vi "Do.vi"(8 "error in (no error)":errorcluster, 10 "Actor in":refnum<class "Actor.lvclass">, 11 "Launch Feature Test View Msg in":refnum<class "Launch Feature Test View Msg.lvclass">) -> (0 "error out":errorcluster, 2 "Actor out":refnum<class "Actor.lvclass">)   [LabVIEW 2023, in "Example Event Actors.lvlib" / "Example Controller Actor.lvlib" / "Launch Feature Test View Msg.lvclass"]
doc: "(<B>Filename</B>: Actor Framework.lvlib:Message.lvclass:Do.vi)\n\nDefines what a message does when it is received by an actor. Generally, a message instructs an actor to invoke one of its methods. By default, this method does nothing. A child class must override it to define behavior. Create a child class by using the Actor Framework Message Maker dialog box."
uses:
  Launch Feature Test View Msg.lvclass
  <vilib>/ActorFramework/Actor/Actor.lvclass
  Example Controller Actor/Example Controller Actor.lvclass
  Launch Feature Test View Msg.lvclass/Launch Feature Test View Msg.ctl
  C:/Projects/Shared Libraries/Event Actors/Examples/Timed Loop Controller/Timed Loop Controller/Timed Loop Controller.lvclass
  C:/Projects/Shared Libraries/Event Actors/Controller Actor/Controller Actor.lvclass
  C:/Program Files/National Instruments/LabVIEW 2023/vi.lib/ActorFramework/Actor/Actor.lvclass
  C:/Projects/Hardware Controller/Source/LSI Hardware Controller/View Interface/IView.lvclass
  C:/Projects/Shared Libraries/Event Actors/Examples/Example Controller Actor/Example Controller Actor/Example Controller Actor.lvclass
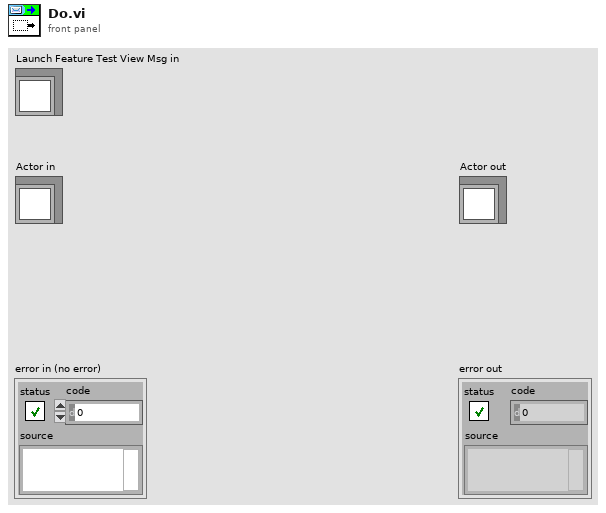
[diagram p1: front panel]
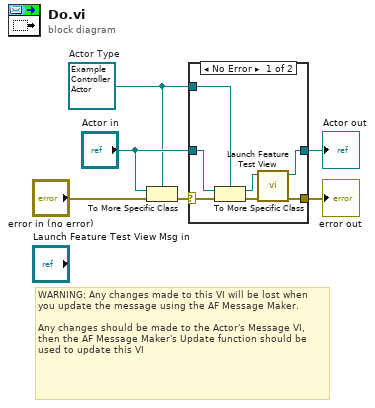
[diagram p0: block diagram]
diagram:
  w1 = refnum<class "Example Controller Actor.lvclass"> refnum  # Actor Type
  # "WARNING: Any changes made to this VI will be lost when you update the message using the AF Message Maker.\n\nAny changes should be made to the Actor's Message VI, then the AF Message Maker's Update function should be used to update this VI"
  n1 = To More Specific Class(target class=w1, reference="Actor in", error in="error in (no error)") -> (error out=w5:errorcluster)  [unwired: 1 out]
  n2 = case shown="No Error" w5 {
    selector: w5 -> [w13 w15]
    tunnel: [w8 w15] -> w4
    tunnel: [w7 w14] -> w3
    tunnel: "Actor in" -> [w12 w14]
    tunnel: w1 -> [w11 _]
    frame No Error {
      n3 = To More Specific Class ("Actor Cast")(target class=w11, reference=w12, error in=w13) -> (specific class reference=w10:refnum<class "Example Controller Actor.lvclass">, error out=w9:errorcluster)
      n4 = call "Launch Feature Test View.vi"("error in (no error)"=w9, "Example Controller Actor in"=w10) -> ("error out"=w8:errorcluster, "Example Controller Actor out"=w7:refnum<class "Example Controller Actor.lvclass">)  [unwired: 8 in]
    }
    frame Error {
    }
  }
  "error out" <- w4
  "Actor out" <- w3
